vi "SubVI Tester.vi"() -> ()   [LabVIEW 2018]
uses:
  Data.ctl
panel:
  in  "Weather Data In":T1={"Units"=enum."", "Current Temperature"=0.0, "Max Temperature"=0.0, "Min Temperature"=0.0, "Warning?"=FALSE, "Warning Text"="No Warning", "Current Windspeed"=0.0, "Max Windspeed"=0.0, "Windspeed Warning?"=FALSE, "Windspeed Warning Text"="No Warning"}
  out "Weather Data Out 2":T1={"Units"=enum."", "Current Temperature"=0.0, "Max Temperature"=0.0, "Min Temperature"=0.0, "Warning?"=FALSE, "Warning Text"="No Warning", "Current Windspeed"=0.0, "Max Windspeed"=0.0, "Windspeed Warning?"=FALSE, "Windspeed Warning Text"="No Warning"}
  in  "Min Temperature":dbl=10.0
  in  "Max Temperature":dbl=30.0
  in  "Stop":bool
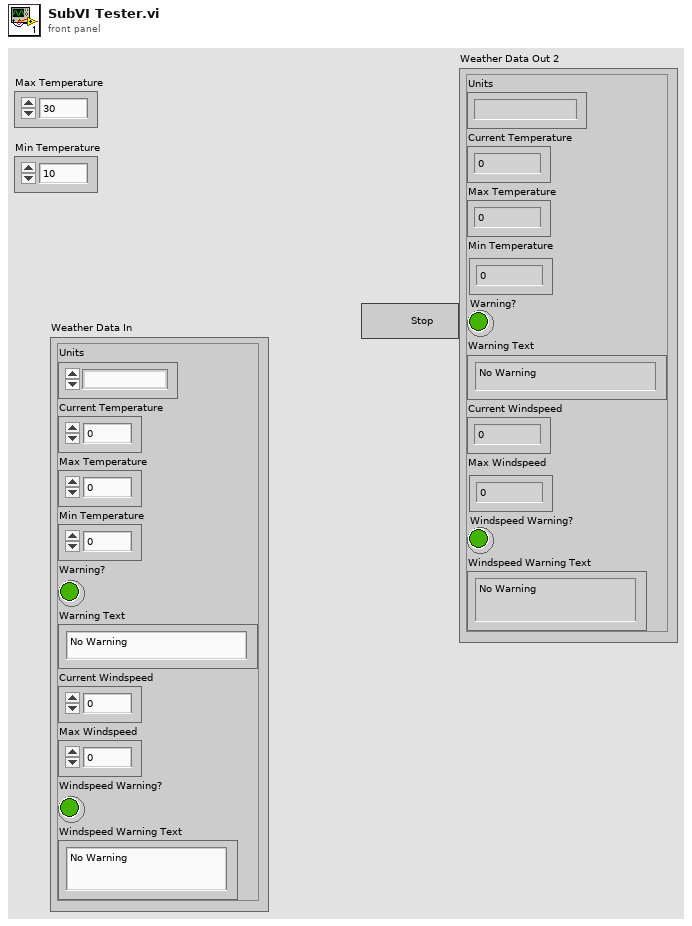
[diagram p1: front panel]
types:
  T1 = typedef "Data.ctl" = cluster{"Units":enum16{"", "Celcius", "Farhrenheit"}, "Current Temperature":dbl, "Max Temperature":dbl, "Min Temperature":dbl, "Warning?":bool, "Warning Text":string, "Current Windspeed":dbl, "Max Windspeed":dbl, "Windspeed Warning?":bool, "Windspeed Warning Text":string}
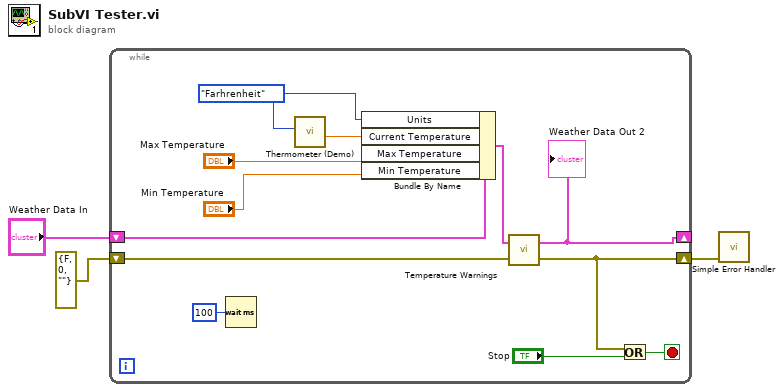
[diagram p0: block diagram]
diagram:
  n1 = while {
    shift-right: [w5] -> w3
    shift-left: errorcluster {"status"=FALSE, "code"=0, "source"=""} ("error in") -> [w6]
    shift-right: [w8] -> _
    shift-left: "Weather Data In" -> [w9]
    stop <- w13 stop-if-true
    w4 = enum16{"", "Celcius", "Farhrenheit"}."Farhrenheit"
    n2 = Wait (ms)(milliseconds to wait=u32 100) -> ()  [unwired: 1 out]
    n3 = call "Thermometer (Demo).vi"("Units (0: Celsius)"=w4) -> ("Temperature Value"=w12:dbl)  [unwired: 10 in]
    n4 = Bundle By Name(cluster=w9, "Units"=w4, "Current Temperature"=w12, "Max Temperature"="Max Temperature", "Min Temperature"="Min Temperature") -> (w7:T1)
    n5 = call "Temperature Warnings.vi"("Error In 2"=w6, "Weather Data In 2"=w7) -> ("Error Out 2"=w5:errorcluster, "Weather Data Out 2"=w8:T1)
    "Weather Data Out 2" <- w8
    n6 = Or(x=w5, y="Stop") -> (x .or. y?=w13:bool)
  }
  n7 = call <vilib>:"Simple Error Handler.vi"("error in (no error)"=w3) -> ()  [unwired: 4 in, 5 out]
